vi "MOVE.vi"(1 "Z":dbl, 2 "Y":dbl, 3 "x":dbl) -> (0 "MOVE COMMAND":string)   [LabVIEW 2014]
panel:
  out "值":i32
  out "子字符串;substring":string
  out "十六进制整型字符串":string
  out "x-y*floor(x/y) 2":dbl
  out "floor(x/y)":dbl
  out "x-y*floor(x/y)":dbl
  out "x*y":dbl
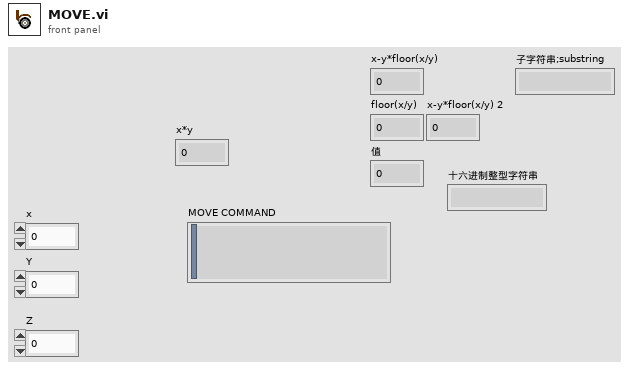
[diagram p1: front panel]
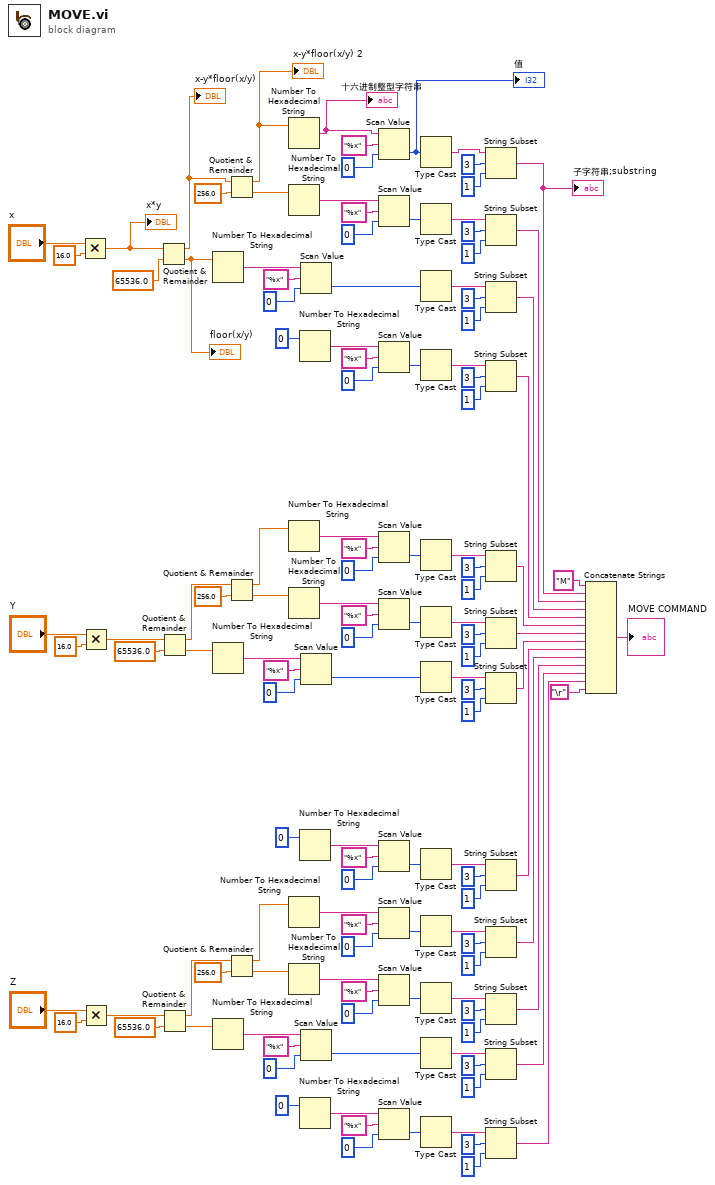
[diagram p0: block diagram]
diagram:
  n1 = Multiply(x="x", y=16.0) -> (x*y=w9:dbl)
  "x*y" <- w9
  n2 = Multiply(x="Y", y=16.0) -> (x*y=w4:dbl)
  n3 = Multiply(x="Z", y=16.0) -> (x*y=w1:dbl)
  n4 = Quotient & Remainder(x=w9, y=65536.0) -> (x-y*floor(x/y)=w26:dbl, floor(x/y)=w22:dbl)
  "x-y*floor(x/y)" <- w26
  "floor(x/y)" <- w22
  n5 = Quotient & Remainder(x=w4, y=65536.0) -> (x-y*floor(x/y)=w20:dbl, floor(x/y)=w11:dbl)
  n6 = Quotient & Remainder(x=w1, y=65536.0) -> (x-y*floor(x/y)=w17:dbl, floor(x/y)=w13:dbl)
  n7 = Number To Hexadecimal String(2:w22) -> (0:w113:string)  [unwired: 1 in]
  n8 = Number To Hexadecimal String(2:w11) -> (0:w81:string)  [unwired: 1 in]
  n9 = Number To Hexadecimal String(2:w13) -> (0:w48:string)  [unwired: 1 in]
  n10 = Quotient & Remainder(x=w26, y=256.0) -> (x-y*floor(x/y)=w23:dbl, floor(x/y)=w24:dbl)
  "x-y*floor(x/y) 2" <- w23
  n11 = Quotient & Remainder(x=w20, y=256.0) -> (x-y*floor(x/y)=w15:dbl, floor(x/y)=w10:dbl)
  n12 = Quotient & Remainder(x=w17, y=256.0) -> (x-y*floor(x/y)=w14:dbl, floor(x/y)=w12:dbl)
  n13 = Number To Hexadecimal String(2:w23) -> (0:w128:string)  [unwired: 1 in]
  "十六进制整型字符串" <- w128
  n14 = Number To Hexadecimal String(2:w24) -> (0:w120:string)  [unwired: 1 in]
  n15 = Number To Hexadecimal String(2:w15) -> (0:w95:string)  [unwired: 1 in]
  n16 = Number To Hexadecimal String(2:w10) -> (0:w88:string)  [unwired: 1 in]
  n17 = Number To Hexadecimal String(2:w14) -> (0:w62:string)  [unwired: 1 in]
  n18 = Number To Hexadecimal String(2:w12) -> (0:w55:string)  [unwired: 1 in]
  n19 = Number To Hexadecimal String(2:0 ("number")) -> (0:w105:string)  [unwired: 1 in]
  n20 = Number To Hexadecimal String(2:0 ("number")) -> (0:w73:string)  [unwired: 1 in]
  n21 = Number To Hexadecimal String(2:0 ("number")) -> (0:w40:string)  [unwired: 1 in]
  n22 = Scan Value(string=w113, format string="%x", default (0 dbl)=0) -> (value=w111:i32)  [unwired: 1 out]
  n23 = Scan Value(string=w81, format string="%x", default (0 dbl)=0) -> (value=w79:i32)  [unwired: 1 out]
  n24 = Scan Value(string=w48, format string="%x", default (0 dbl)=0) -> (value=w46:i32)  [unwired: 1 out]
  n25 = Scan Value(string=w128, format string="%x", default (0 dbl)=0) -> (value=w126:i32)  [unwired: 1 out]
  "值" <- w126
  n26 = Scan Value(string=w120, format string="%x", default (0 dbl)=0) -> (value=w118:i32)  [unwired: 1 out]
  n27 = Scan Value(string=w105, format string="%x", default (0 dbl)=0) -> (value=w103:i32)  [unwired: 1 out]
  n28 = Scan Value(string=w95, format string="%x", default (0 dbl)=0) -> (value=w93:i32)  [unwired: 1 out]
  n29 = Scan Value(string=w88, format string="%x", default (0 dbl)=0) -> (value=w86:i32)  [unwired: 1 out]
  n30 = Scan Value(string=w73, format string="%x", default (0 dbl)=0) -> (value=w71:i32)  [unwired: 1 out]
  n31 = Scan Value(string=w62, format string="%x", default (0 dbl)=0) -> (value=w60:i32)  [unwired: 1 out]
  n32 = Scan Value(string=w55, format string="%x", default (0 dbl)=0) -> (value=w53:i32)  [unwired: 1 out]
  n33 = Scan Value(string=w40, format string="%x", default (0 dbl)=0) -> (value=w38:i32)  [unwired: 1 out]
  n34 = Type Cast(x=w126) -> (*(type *) &x=w122:string)  [unwired: 1 in]
  n35 = Type Cast(x=w118) -> (*(type *) &x=w114:string)  [unwired: 1 in]
  n36 = Type Cast(x=w111) -> (*(type *) &x=w107:string)  [unwired: 1 in]
  n37 = Type Cast(x=w103) -> (*(type *) &x=w99:string)  [unwired: 1 in]
  n38 = Type Cast(x=w93) -> (*(type *) &x=w89:string)  [unwired: 1 in]
  n39 = Type Cast(x=w86) -> (*(type *) &x=w82:string)  [unwired: 1 in]
  n40 = Type Cast(x=w79) -> (*(type *) &x=w75:string)  [unwired: 1 in]
  n41 = Type Cast(x=w71) -> (*(type *) &x=w67:string)  [unwired: 1 in]
  n42 = Type Cast(x=w60) -> (*(type *) &x=w56:string)  [unwired: 1 in]
  n43 = Type Cast(x=w53) -> (*(type *) &x=w49:string)  [unwired: 1 in]
  n44 = Type Cast(x=w46) -> (*(type *) &x=w42:string)  [unwired: 1 in]
  n45 = Type Cast(x=w38) -> (*(type *) &x=w34:string)  [unwired: 1 in]
  n46 = String Subset(string=w122, offset (0)=3, length (rest)=1 ("length (rest)")) -> (substring=w121:string)
  "子字符串;substring" <- w121
  n47 = String Subset(string=w114, offset (0)=3, length (rest)=1 ("length (rest)")) -> (substring=w98:string)
  n48 = String Subset(string=w107, offset (0)=3, length (rest)=1 ("length (rest)")) -> (substring=w97:string)
  n49 = String Subset(string=w99, offset (0)=3, length (rest)=1 ("length (rest)")) -> (substring=w96:string)
  n50 = String Subset(string=w89, offset (0)=3, length (rest)=1 ("length (rest)")) -> (substring=w66:string)
  n51 = String Subset(string=w82, offset (0)=3, length (rest)=1 ("length (rest)")) -> (substring=w65:string)
  n52 = String Subset(string=w75, offset (0)=3, length (rest)=1 ("length (rest)")) -> (substring=w64:string)
  n53 = String Subset(string=w67, offset (0)=3, length (rest)=1 ("length (rest)")) -> (substring=w63:string)
  n54 = String Subset(string=w56, offset (0)=3, length (rest)=1 ("length (rest)")) -> (substring=w33:string)
  n55 = String Subset(string=w49, offset (0)=3, length (rest)=1 ("length (rest)")) -> (substring=w32:string)
  n56 = String Subset(string=w42, offset (0)=3, length (rest)=1 ("length (rest)")) -> (substring=w31:string)
  n57 = String Subset(string=w34, offset (0)=3, length (rest)=1 ("length (rest)")) -> (substring=w30:string)
  n58 = Concatenate Strings("M" ("string"), w121, w98, w97, w96, w66, w65, w64, w63, w33, w32, w31, w30, "\r") -> (→"MOVE COMMAND":string)
